vi "New.vi"(4 "Inverted":bool, 6 "Delimiters":T1={"Close"="}}", "Open"="{{"}, 8 "Error In":errorcluster, 11 "Key":string) -> (0 "Error Out":errorcluster, 3 "Section":refnum<class "Section.lvclass">)   [LabVIEW 2018, in "Toolkit.lvlib" / "Nodes.lvlib" / "Section.lvclass"]
doc: "Creates a new Section node that represents a Mustache Section or Inverted Section tag in a parsed template."
uses:
  Section.lvclass
  Type Definitions/Delimiters.ctl
  Section.lvclass/Section.ctl
  Toolkit.lvlib
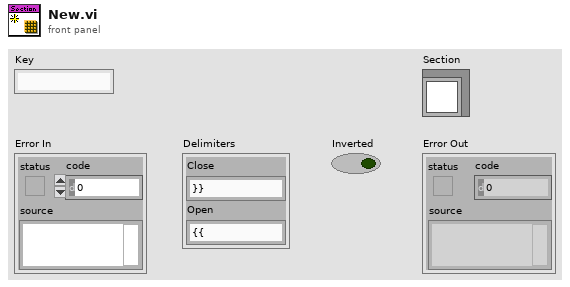
[diagram p1: front panel]
types:
  T1 = typedef "Toolkit.lvlib/Delimiters.ctl" = cluster{"Close":string, "Open":string}
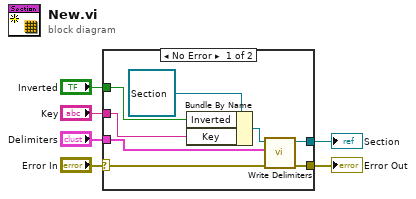
[diagram p0: block diagram]
diagram:
  n1 = case shown="No Error" "Error In" {
    selector: "Error In" -> [w8 w15]
    tunnel: "Key" -> [w14 _]
    tunnel: "Inverted" -> [w13 _]
    tunnel: [w10 _] -> w4
    tunnel: [w9 w15] -> w3
    tunnel: "Delimiters" -> [w7 _]
    frame No Error {
      n2 = Bundle By Name(cluster=refnum<class "Section.lvclass"> refnum ("Toolkit.lvlib:Nodes.lvlib:Section.lvclass"), "Inverted"=w13, "Key"=w14) -> (w11:refnum<class "Section.lvclass">)
      n3 = call-dynamic "Write Delimiters.vi"("Error In"=w8, "Delimiters"=w7, "Node In"=w11) -> ("Error Out"=w9:errorcluster, "Node Out"=w10:refnum<class "Section.lvclass">)  [unwired: 7 in]
    }
    frame Error {
    }
  }
  "Section" <- w4
  "Error Out" <- w3
